vi "DrawSwitches.vi"(8 "error in (no error)":errorcluster, 11 "SnakeGame in":refnum<class "SnakeGame.lvclass">) -> (0 "error out":errorcluster, 3 "SnakeGame out":refnum<class "SnakeGame.lvclass">)   [LabVIEW 2019, in "RT_Game.lvlib" / "SnakeGame.lvclass"]
uses:
  SnakeGame.lvclass
  C:/Users/FreshBob/Dropbox/VIs/myRIO_GameConsole/RT/RT_Game/Game/Game.lvclass
  SnakeGame.lvclass/SnakeGame.ctl
  GameObject/GameObject.lvclass/GameObject.ctl
  PongSwitch/SnakeSwitch.lvclass/SnakeSwitch.ctl
  GameObject/Read position.vi
  PongSwitch/Read Tilecode.vi
  GameObject/Read IsActive.vi
  PongSwitch/SnakeSwitch.lvclass
  C:/Users/FreshBob/Dropbox/VIs/myRIO_GameConsole/RT/RT_Game/GameObject/GameObject.lvclass
  Game/Game.lvclass
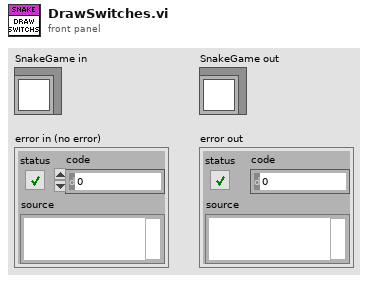
[diagram p1: front panel]
types:
  T1 = typedef "RT_Game.lvlib/Game.lvclass/Coordinate.ctl" = cluster{"x":dbl, "y":dbl}
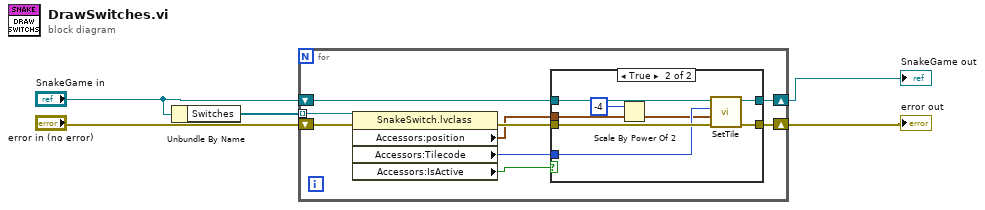
[diagram p0: block diagram]
diagram:
  n1 = Unbundle By Name("SnakeGame in") -> ("Switches"=w2:refnum<class "SnakeSwitch.lvclass">[])
  n2 = for {
    shift-right: [w14] -> w1
    shift-left: "SnakeGame in" -> [w13]
    shift-right: [w12] -> w5
    shift-left: "error in (no error)" -> [w11]
    tunnel: w2 -> [w9] mode=indexing
    n3 = property class="SnakeSwitch.lvclass"(reference=w9, error in=w11) -> (error out=w10:errorcluster, "Accessors:position"=w8:T1, "Accessors:Tilecode"=w7:u32, "Accessors:IsActive"=w6:bool)  [unwired: 1 out]
    n4 = case shown="True" w6 {
      tunnel: [w16 w24] -> w14
      tunnel: w13 -> [w16 w23]
      tunnel: [w15 w22] -> w12
      tunnel: w10 -> [w15 w21]
      tunnel: w8 -> [_ w20]
      tunnel: w7 -> [_ w19]
      frame False {
      }
      frame True {
        n5 = Scale By Power Of 2(n=i16 -4, x=w20) -> (x*2^n=w18:T1)
        n6 = call "SetTile.vi"("error in (no error)"=w21, "Coordinates"=w18, "TileNumber"=w19, "Game in"=w23) -> ("error out"=w22:errorcluster, "Game out"=w24:refnum<class "SnakeGame.lvclass">)  [unwired: 6 in]
      }
    }
  }
  "SnakeGame out" <- w1
  "error out" <- w5
